vi "DriversStationCodeNew.vi"(9 "Left":bool, 11 "Image Out":T1) -> (3 "Image Out 2":T1)   [LabVIEW 2011]
uses:
  <vilib>/vision/Image Controls.llb/IMAQ Image.ctl
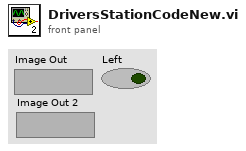
[diagram p1: front panel]
types:
  T1 = typedef "IMAQ Image.ctl" = refnum<image>
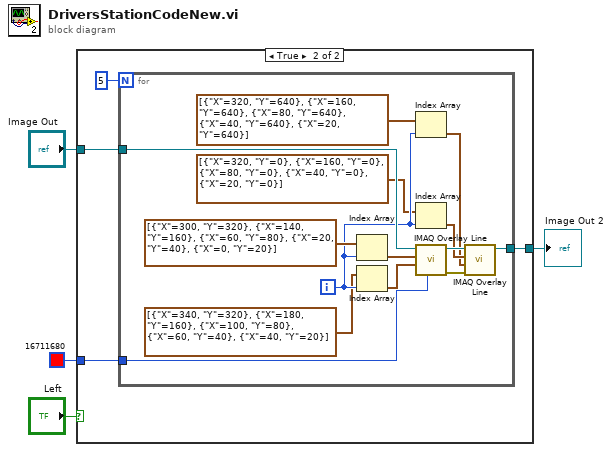
[diagram p0: block diagram]
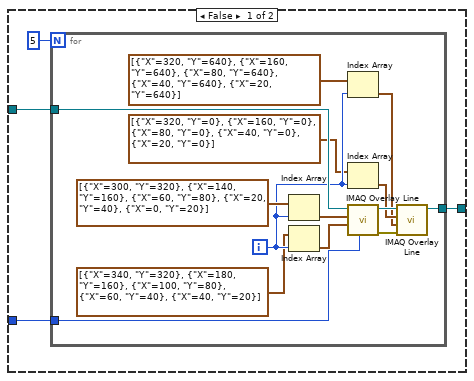
[diagram p2: hidden frame]
diagram:
  n1 = case shown="True" "Left" {
    tunnel: u32 16711680 ("Color") -> [w6 w25]
    tunnel: "Image Out" -> [w5 w24]
    tunnel: [w7 w23] -> w2
    frame False {
      n2 = for {
        N: 5 -> [_]
        tunnel: w5 -> [w22]
        tunnel: w6 -> [w21]
        tunnel: [w20] -> w7
        i -> [w16]
        n3 = Index Array(array=cluster{"X":i32, "Y":i32}[] [{"X"=300, "Y"=320}, {"X"=140, "Y"=160}, {"X"=60, "Y"=80}, {"X"=20, "Y"=40}, {"X"=0, "Y"=20}], index=w16) -> (element=w12:cluster{"X":i32, "Y":i32})
        n4 = Index Array(array=cluster{"X":i32, "Y":i32}[] [{"X"=340, "Y"=320}, {"X"=180, "Y"=160}, {"X"=100, "Y"=80}, {"X"=60, "Y"=40}, {"X"=40, "Y"=20}], index=w16) -> (element=w11:cluster{"X":i32, "Y":i32})
        n5 = Index Array(array=cluster{"X":i32, "Y":i32}[] [{"X"=320, "Y"=640}, {"X"=160, "Y"=640}, {"X"=80, "Y"=640}, {"X"=40, "Y"=640}, {"X"=20, "Y"=640}], index=w16) -> (element=w9:cluster{"X":i32, "Y":i32})
        n6 = Index Array(array=cluster{"X":i32, "Y":i32}[] [{"X"=320, "Y"=0}, {"X"=160, "Y"=0}, {"X"=80, "Y"=0}, {"X"=40, "Y"=0}, {"X"=20, "Y"=0}], index=w16) -> (element=w10:cluster{"X":i32, "Y":i32})
        n7 = call "IMAQ Overlay Line"("Color"=w21, "End Point"=w11, "Start Point"=w12, "Image"=w22) -> ("error out"=w18:errorcluster, "Image Out"=w19:T1)  [unwired: 6 in]
        n8 = call "IMAQ Overlay Line"("error in (no error)"=w18, "End Point"=w9, "Start Point"=w10, "Image"=w19) -> ("Image Out"=w20:T1)  [unwired: 6 in, 1 out]
      }
    }
    frame True {
      n9 = for {
        N: 5 -> [_]
        tunnel: w24 -> [w40]
        tunnel: w25 -> [w39]
        tunnel: [w38] -> w23
        i -> [w34]
        n10 = Index Array(array=cluster{"X":i32, "Y":i32}[] [{"X"=300, "Y"=320}, {"X"=140, "Y"=160}, {"X"=60, "Y"=80}, {"X"=20, "Y"=40}, {"X"=0, "Y"=20}], index=w34) -> (element=w30:cluster{"X":i32, "Y":i32})
        n11 = Index Array(array=cluster{"X":i32, "Y":i32}[] [{"X"=340, "Y"=320}, {"X"=180, "Y"=160}, {"X"=100, "Y"=80}, {"X"=60, "Y"=40}, {"X"=40, "Y"=20}], index=w34) -> (element=w29:cluster{"X":i32, "Y":i32})
        n12 = Index Array(array=cluster{"X":i32, "Y":i32}[] [{"X"=320, "Y"=640}, {"X"=160, "Y"=640}, {"X"=80, "Y"=640}, {"X"=40, "Y"=640}, {"X"=20, "Y"=640}], index=w34) -> (element=w27:cluster{"X":i32, "Y":i32})
        n13 = Index Array(array=cluster{"X":i32, "Y":i32}[] [{"X"=320, "Y"=0}, {"X"=160, "Y"=0}, {"X"=80, "Y"=0}, {"X"=40, "Y"=0}, {"X"=20, "Y"=0}], index=w34) -> (element=w28:cluster{"X":i32, "Y":i32})
        n14 = call "IMAQ Overlay Line"("Color"=w39, "End Point"=w29, "Start Point"=w30, "Image"=w40) -> ("error out"=w36:errorcluster, "Image Out"=w37:T1)  [unwired: 6 in]
        n15 = call "IMAQ Overlay Line"("error in (no error)"=w36, "End Point"=w27, "Start Point"=w28, "Image"=w37) -> ("Image Out"=w38:T1)  [unwired: 6 in, 1 out]
      }
    }
  }
  "Image Out 2" <- w2
